vi "Motor Status Wait X.vi"(3 "Error In":errorcluster, 5 "Reference In":refnum<class "_Controller.lvclass">) -> (0 "Error Out":errorcluster, 2 "Reference Out":refnum<class "_Controller.lvclass">)   [LabVIEW 2020]
doc: "Waits for motor X to be in idle (i.e. not moving). This is done to ensure motor X has completed any neccessary movement before sending the next command. Otherwise a pulsing error is obtained.\n\nArgs:\n\nReference In: Incoming communication (reference) between LabView and the scanning rig controller\nError In: Checks for any errors with the incoming communication (reference)\n\nReturns:\n\nReference Out: Output communnication (reference) between LabView and controller\nError Out: Checks for any error with output communication (reference)"
uses:
  <instrlib>/Arcus Ethernet Driver 1.0.0/ArcusEthernetComm/classes/Controller/_Controller.lvclass
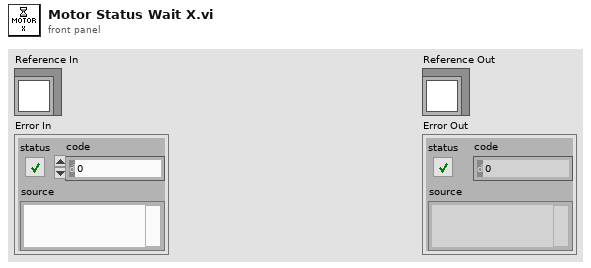
[diagram p1: front panel]
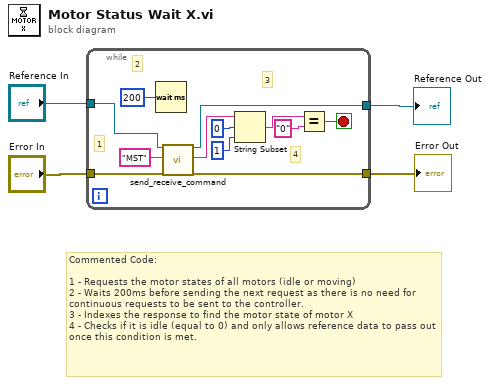
[diagram p0: block diagram]
diagram:
  # "Commented Code:\n\n1 - Requests the motor states of all motors (idle or moving)\n2 - Waits 200ms before sending the next request as there is no need for continuous requests to be sent to the controller. \n3 - Indexes the response to find the motor state of motor X\n4 - Checks if it is idle (equal to 0) and only allows reference data to pass out once this condition is met."
  n1 = while {
    tunnel: "Reference In" -> [w7]
    tunnel: "Error In" -> [w6]
    tunnel: [w8] -> w2
    tunnel: [w5] -> w1
    stop <- w9 stop-if-true
    # "4"
    # "3"
    # "2"
    # "1"
    n2 = Wait (ms)(milliseconds to wait=u32 200) -> ()  [unwired: 1 out]
    n3 = call <instrlib>:"send_receive_command.vi"("reference (in)"=w7, "ASCII Command (in)"="MST", "error in (no error)"=w6) -> ("reference (out)"=w8:refnum<class "_Controller.lvclass">, "response (out)"=w12:string, "error out"=w5:errorcluster)  [unwired: 12 in, 2 out]
    n4 = String Subset(string=w12, offset (0)=0, length (rest)=1 ("length (rest)")) -> (substring=w11:string)
    n5 = Equal?(x=w11, y="0") -> (x = y?=w9:bool)
  }
  "Reference Out" <- w2
  "Error Out" <- w1
